vi "add_empty_row_to_ItemNames.vi"(7 "multicolumn_listbox_reference_in":refnum<vi>, 11 "ItemNames_in":string[][](array[string])) -> (3 "ItemNames_out":string[][](array[string]))   [LabVIEW 2019]
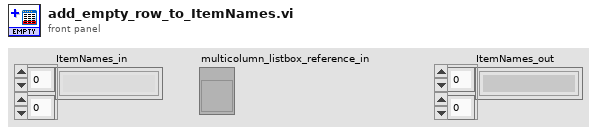
[diagram p1: front panel]
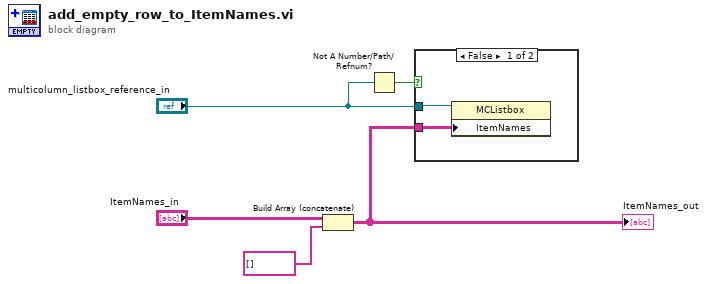
[diagram p0: block diagram]
diagram:
  n1 = Build Array (concatenate)("ItemNames_in", string[] []) -> (w1:string[][])
  "ItemNames_out" <- w1
  n2 = Not A Number/Path/Refnum?(number/path/refnum="multicolumn_listbox_reference_in") -> (NaN/Path/Refnum?=w3:bool)
  n3 = case shown="False" w3 {
    tunnel: "multicolumn_listbox_reference_in" -> [w7 _]
    tunnel: w1 -> [w6 _]
    frame False {
      n4 = property class="MCListbox"(reference=w7, "ItemNames"=w6) -> ()  [unwired: 1 in, 2 out]
    }
    frame True {
    }
  }
